vi "Read Forward Power.vi"(8 "error in (no error)":errorcluster, 10 "average (false)":bool, 11 "VI Probe in":refnum<class "PL MKS VI Probe.lvclass">) -> (0 "error out":errorcluster, 2 "Pfwd, W":dbl, 3 "VI Probe out":refnum<class "PL MKS VI Probe.lvclass">)   [LabVIEW 2015, in "PL MKS VI Probe.lvclass"]
doc: "Reads forward power."
uses:
  PL MKS VI Probe.lvclass
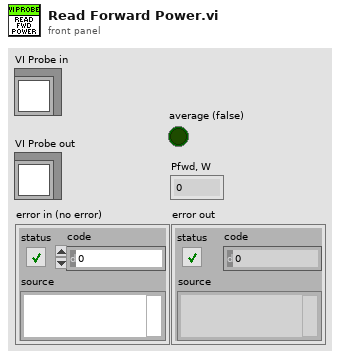
[diagram p1: front panel]
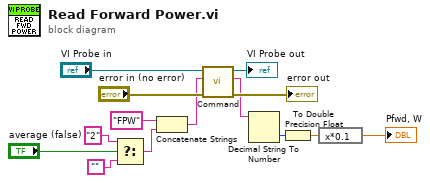
[diagram p0: block diagram]
diagram:
  n1 = Select(t="2", s="average (false)", f="") -> (s? t:f=w3:string)
  n2 = Concatenate Strings("FPW" ("format string"), w3) -> (w4:string)
  n3 = call "Command.vi"("error in (no error)"="error in (no error)", "command"=w4, "VI Probe in"="VI Probe in") -> ("error out"=→"error out":errorcluster, "response data"=w10:string, "VI Probe out"=→"VI Probe out":refnum<class "PL MKS VI Probe.lvclass">)  [unwired: 6 in]
  n4 = Decimal String To Number(string=w10) -> (number=w9:i32)  [unwired: 2 in, 1 out]
  n5 = To Double Precision Float(number=w9) -> (double precision float=w2:dbl)
  n6 = expression code="x*0.1"(w2) -> (→"Pfwd, W":dbl)
